vi "Optimization.vi"(0 "GoalAngle0":dbl format="%#_13g", 1 "Az0":dbl format="%#_13g", 2 "GoalAngle1":dbl format="%#_13g", 3 "Az1":dbl format="%#_13g", 4 "GoalAngle2":dbl format="%#_13g", 5 "Az2":dbl format="%#_13g", 6 "GoalAngle3":dbl format="%#_13g", 7 "Az3":dbl format="%#_13g", 8 "PID gains":T1={"proportional gain (Kc)"=0.008, "integral time (Ti, min)"=0.0, "derivative time (Td, min)"=0.0} {"derivative time (Td, min)" format="%.3f"; "integral time (Ti, min)" format="%.3f"; "proportional gain (Kc)" format="%.3f"}) -> (20 "A0":dbl format="%.2f", 21 "Flip0":bool, 22 "A1":dbl format="%.2f", 23 "Flip1":bool, 24 "A2":dbl format="%.2f", 25 "Flip2":bool, 26 "A3":dbl format="%.2f", 27 "Flip3":bool)   [LabVIEW 2020]
uses:
  <vilib>/addons/control/pid/NI_PID_pid.lvlib
  <vilib>/addons/control/pid/pid.llb/PID (DBL).vi
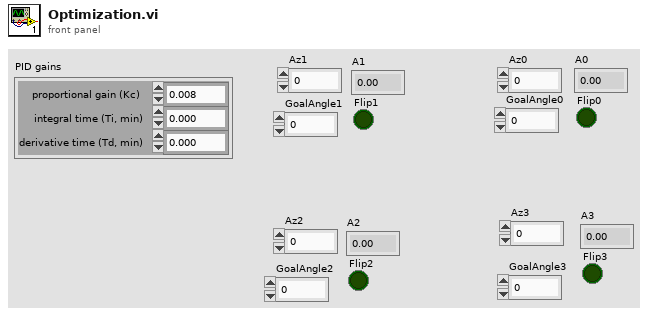
[diagram p1: front panel]
types:
  T1 = cluster{"proportional gain (Kc)":dbl, "integral time (Ti, min)":dbl, "derivative time (Td, min)":dbl}
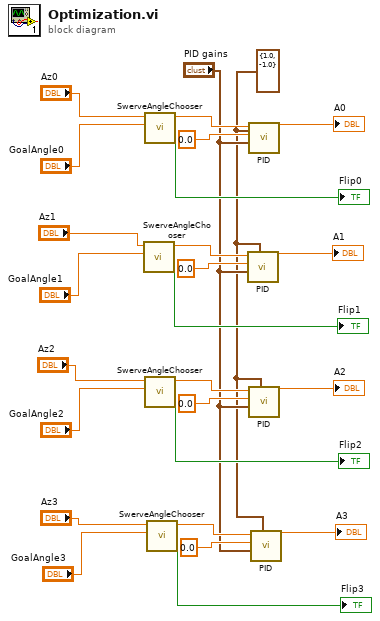
[diagram p0: block diagram]
diagram:
  w5 = cluster{"output high":dbl, "output low":dbl} {"output high"=1.0, "output low"=-1.0} ("output range")
  n1 = call "SwerveAngleChooser.vi"("Goal Angle (deg) [-180,+180]"="GoalAngle1", "Current Angle (deg) [-180,+180]"="Az1") -> ("Flip Drive Motor Direction"=→"Flip1":bool, "Angular Distance (deg)"=w18:dbl)  [unwired: 8 in]
  n2 = call "SwerveAngleChooser.vi"("Goal Angle (deg) [-180,+180]"="GoalAngle0", "Current Angle (deg) [-180,+180]"="Az0") -> ("Flip Drive Motor Direction"=→"Flip0":bool, "Angular Distance (deg)"=w25:dbl)  [unwired: 8 in]
  n3 = call "SwerveAngleChooser.vi"("Goal Angle (deg) [-180,+180]"="GoalAngle2", "Current Angle (deg) [-180,+180]"="Az2") -> ("Flip Drive Motor Direction"=→"Flip2":bool, "Angular Distance (deg)"=w15:dbl)  [unwired: 8 in]
  n4 = call "SwerveAngleChooser.vi"("Goal Angle (deg) [-180,+180]"="GoalAngle3", "Current Angle (deg) [-180,+180]"="Az3") -> ("Flip Drive Motor Direction"=→"Flip3":bool, "Angular Distance (deg)"=w8:dbl)  [unwired: 8 in]
  n5 = call-poly <vilib>:"PID.vi"("output range"=w5, "PID gains"="PID gains", "process variable"=0.0, "setpoint"=w18) -> ("output"=→"A1":dbl)  [unwired: 6 in, 1 out]
  n6 = call-poly <vilib>:"PID.vi"("output range"=w5, "PID gains"="PID gains", "process variable"=0.0, "setpoint"=w25) -> ("output"=→"A0":dbl)  [unwired: 6 in, 1 out]
  n7 = call-poly <vilib>:"PID.vi"("output range"=w5, "PID gains"="PID gains", "process variable"=0.0, "setpoint"=w15) -> ("output"=→"A2":dbl)  [unwired: 6 in, 1 out]
  n8 = call-poly <vilib>:"PID.vi"("output range"=w5, "PID gains"="PID gains", "process variable"=0.0, "setpoint"=w8) -> ("output"=→"A3":dbl)  [unwired: 6 in, 1 out]
